vi "CvrtGrp2GXML.vi"(8 "error in (no error)":errorcluster, 11 "ChanGroups in":refnum<class "ChanGrp.lvclass">[](array[class])) -> (0 "error out":errorcluster, 1 "GXML Chans Oout":string[](array[string]), 3 "ChanGroups out":T1)   [LabVIEW 2018, in "Configuration Grandmaster.lvlib" / "ChanGrp.lvclass"]
uses:
  ChanGrp.lvclass
  Custom Ctrls/Master CfgXML/ge_XMLHdr_ChanGroups.ctl
  Custom Ctrls/Master Cfg/ge_GrpHdr.ctl
  Custom Ctrls/ge_MeasType.ctl
  ChanGrp.lvclass/ChanGrp.ctl
  Measurement Type Defs/VoltGroup.ctl
  Measurement Type Defs/VoltChan.ctl
  Measurements/Class Channel/ChanProps_TD.ctl
  Measurements/Class Voltage/VoltProps_TD.ctl
  Measurements/Class Voltage/Voltage.lvclass
  Measurement Type Defs/FreqGroup.ctl
  Measurement Type Defs/FreqChan.ctl
  Measurements/Class Frequency/FreqProps_TD.ctl
  Measurements/Class Frequency/Frequency.lvclass
  Measurement Type Defs/TachGroup.ctl
  Measurement Type Defs/TachChan.ctl
  Measurements/Class Tachometer/TachProps_TD.ctl
  Measurements/Class Tachometer/Tachometer.lvclass
  Measurement Type Defs/DynGroup.ctl
  Measurement Type Defs/DyanChan.ctl
  Measurements/Class Dynamic/DynamicProps_TD.ctl
  Measurements/Class Dynamic/Dynamic.lvclass
  Measurement Type Defs/StrainGroup.ctl
  Measurement Type Defs/StrainChan.ctl
  Measurements/Class Strain/StrainProps_TD.ctl
  Measurements/Class Strain/Strain.lvclass
  Measurement Type Defs/ThrmcplGroup.ctl
  Measurement Type Defs/ThrmcplChan.ctl
  Measurements/Class Thermocouple/ThrmcplProps_TD.ctl
  Measurements/Class Thermocouple/Thermocouple.lvclass
  Measurement Type Defs/RTDGroup.ctl
  Measurement Type Defs/RTDChan.ctl
  Measurements/Class RTD/RTDProps_TD.ctl
  Measurements/Class RTD/RTD.lvclass
  Measurement Type Defs/CurrentGroup.ctl
  Measurement Type Defs/CurrentChan.ctl
  Measurements/Class Current/CurrentProps_TD.ctl
  Measurements/Class Current/Current.lvclass
  Measurement Type Defs/ResGroup.ctl
  Measurement Type Defs/ResChan.ctl
  Measurements/Class Ressistance/ResProps_TD.ctl
  Measurements/Class Ressistance/Resistance.lvclass
  Measurements/Class Channel/Channel.lvclass
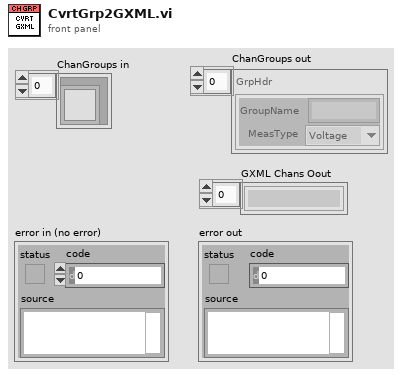
[diagram p1: front panel]
types:
  T1 = typedef "ge_XMLHdr_ChanGroups.ctl" = T2[]
  T2 = typedef "ge_GrpHdr.ctl" = cluster{"GroupName":string, "MeasType":T3}
  T3 = typedef "ge_MeasType.ctl" = enum16{"Voltage", "Frequency", "Tachometer", "Dynamic", "Thermocouple", "RTD", "Strain", "Current", "Resistance"}
  T4 = typedef "Configuration Grandmaster.lvlib/ChanGrp.lvclass/VoltGroup.ctl" = cluster{"GroupName":string, "MeasType":T3, "GroupMems":T5[]}
  T5 = typedef "Configuration Grandmaster.lvlib/ChanGrp.lvclass/VoltChan.ctl" = cluster{"ChanHdr":T6, "VoltChanCfg":T7}
  T6 = typedef "Measurement Channels.lvlib/Channel.lvclass/ChanProps_TD.ctl" = cluster{"ChanName":string, "ModbusAddr":string, "ToModBus":bool, "Alias":string, "Device":string, "Unit_EU":string, "Scale":dbl, "Offset":dbl}
  T7 = typedef "Measurement Channels.lvlib/Voltage.lvclass/VoltProps_TD.ctl" = cluster{"VRange":dbl, "Term Cfg":u16, "Coupling":u16}
  T8 = typedef "Configuration Grandmaster.lvlib/ChanGrp.lvclass/FreqGroup.ctl" = cluster{"GroupName":string, "MeasType":T3, "GroupMems":T9[]}
  T9 = typedef "Configuration Grandmaster.lvlib/ChanGrp.lvclass/FreqChan.ctl" = cluster{"ChanHdr":T6, "VoltChanCfg":T7, "FreqChanCfg":T10}
  T10 = typedef "Measurement Channels.lvlib/Frequency.lvclass/FreqProps_TD.ctl" = cluster{"Thresh":dbl, "Slope":u16, "Min EU":dbl}
  T11 = typedef "Configuration Grandmaster.lvlib/ChanGrp.lvclass/TachGroup.ctl" = cluster{"GroupName":string, "MeasType":T3, "GroupMems":T12[]}
  T12 = typedef "Configuration Grandmaster.lvlib/ChanGrp.lvclass/TachChan.ctl" = cluster{"ChanHdr":T6, "VoltChanCfg":T7, "FreqChanCfg":T10, "TachChanCfg":T13}
  T13 = typedef "Measurement Channels.lvlib/Tachometer.lvclass/TachProps_TD.ctl" = cluster{"PPR":dbl}
  T14 = typedef "Configuration Grandmaster.lvlib/ChanGrp.lvclass/DynGroup.ctl" = cluster{"GroupName":string, "MeasType":T3, "GroupMems":T15[]}
  T15 = typedef "Configuration Grandmaster.lvlib/ChanGrp.lvclass/DyanChan.ctl" = cluster{"ChanHdr":T6, "VoltChanCfg":T7, "DynChanCfg":T16}
  T16 = typedef "Measurement Channels.lvlib/Dynamic.lvclass/DynamicProps_TD.ctl" = cluster{"Sensitivity":dbl, "Iex":dbl, "dB":bool, "dB Ref":dbl, "Cal Mag":dbl, "Cal Units":u16}
  T17 = typedef "Configuration Grandmaster.lvlib/ChanGrp.lvclass/StrainGroup.ctl" = cluster{"GroupName":string, "MeasType":T3, "GroupMems":T18[]}
  T18 = typedef "Configuration Grandmaster.lvlib/ChanGrp.lvclass/StrainChan.ctl" = cluster{"ChanHdr":T6, "StrainChanCfg":T19}
  T19 = typedef "Measurement Channels.lvlib/Strain.lvclass/StrainProps_TD.ctl" = cluster{"Strain Mode":u16, "Vex":dbl, "Bridge Type":u16, "GF":dbl, "Gauge Res":i32, "Poisson":dbl, "Lead Res":dbl, "Init uStrain":dbl, "GAF":dbl, "Approx Max":dbl, "Approx Min":dbl}
  T20 = typedef "Configuration Grandmaster.lvlib/ChanGrp.lvclass/ThrmcplGroup.ctl" = cluster{"GroupName":string, "MeasType":T3, "GroupMems":T21[]}
  T21 = typedef "Configuration Grandmaster.lvlib/ChanGrp.lvclass/ThrmcplChan.ctl" = cluster{"ChanHdr":T6, "ThrmcplChanCfg":T22}
  T22 = typedef "Measurement Channels.lvlib/Thermocouple.lvclass/ThrmcplProps_TD.ctl" = cluster{"Units":u16, "Type":u16, "cjc source":u16, "cjc val":dbl, "Approx Max":dbl, "Approx Min":dbl}
  T23 = typedef "Configuration Grandmaster.lvlib/ChanGrp.lvclass/RTDGroup.ctl" = cluster{"GroupName":string, "MeasType":T3, "GroupMems":T24[]}
  T24 = typedef "Configuration Grandmaster.lvlib/ChanGrp.lvclass/RTDChan.ctl" = cluster{"ChanHdr":T6, "RTDChanCfg":T25}
  T25 = typedef "Measurement Channels.lvlib/RTD.lvclass/RTDProps_TD.ctl" = cluster{"Ro":u16, "Units":u16, "Type":u16, "WireCfg":u16, "Approx Max":dbl, "Approx Min":dbl}
  T26 = typedef "Configuration Grandmaster.lvlib/ChanGrp.lvclass/CurrentGroup.ctl" = cluster{"GroupName":string, "MeasType":T3, "GroupMems":T27[]}
  T27 = typedef "Configuration Grandmaster.lvlib/ChanGrp.lvclass/CurrentChan.ctl" = cluster{"ChanHdr":T6, "CurrentChanCfg":T28}
  T28 = typedef "CurrentProps_TD.ctl" = cluster{"IRange":dbl}
  T29 = typedef "Configuration Grandmaster.lvlib/ChanGrp.lvclass/ResGroup.ctl" = cluster{"GroupName":string, "MeasType":T3, "GroupMems":T30[]}
  T30 = typedef "Configuration Grandmaster.lvlib/ChanGrp.lvclass/ResChan.ctl" = cluster{"ChanHdr":T6, "ResChanCfg":T31}
  T31 = typedef "Measurement Channels.lvlib/Resistance.lvclass/ResProps_TD.ctl" = cluster{"ORange":u16, "WireCfg":u16}
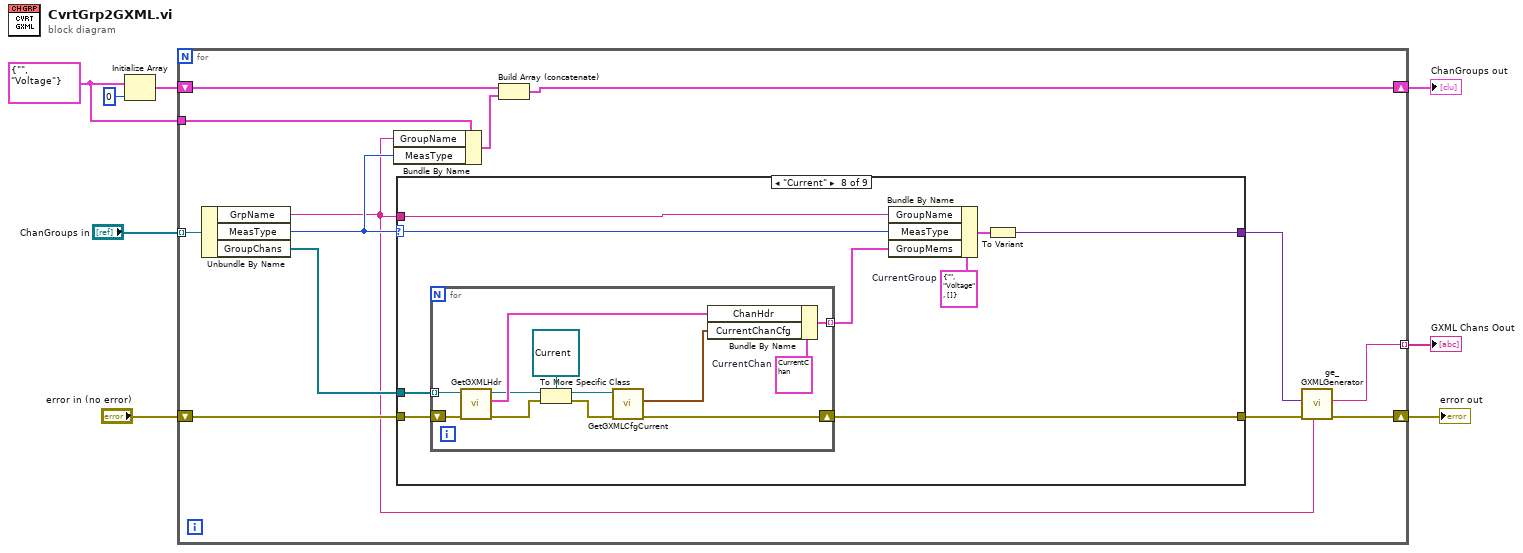
[diagram p0: block diagram]
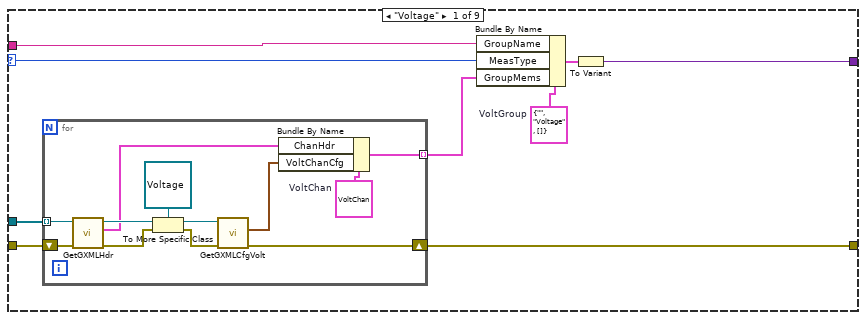
[diagram p2: hidden frame]
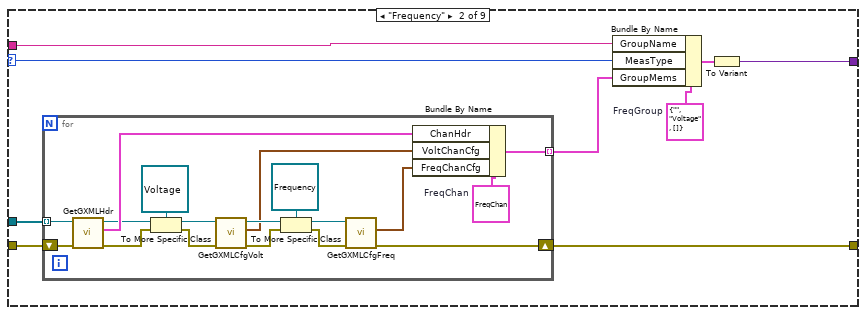
[diagram p3: hidden frame]
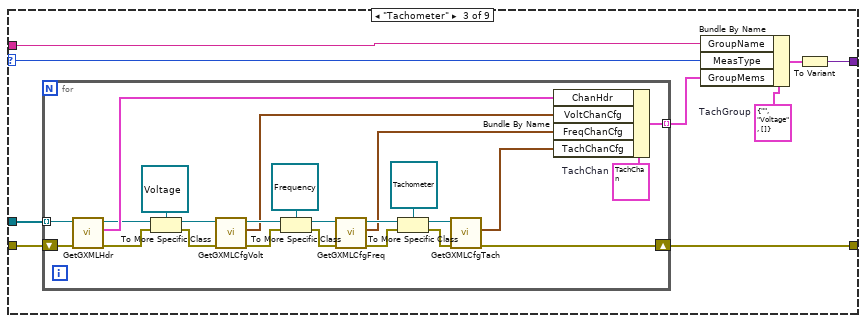
[diagram p4: hidden frame]
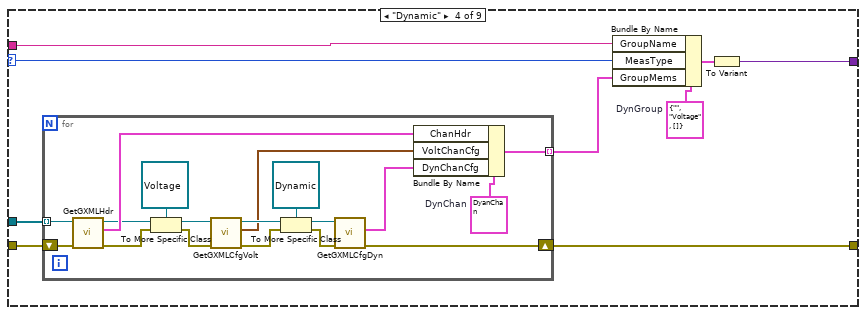
[diagram p5: hidden frame]
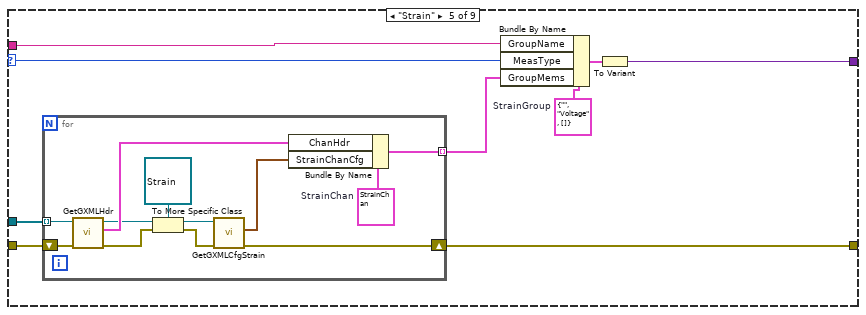
[diagram p6: hidden frame]
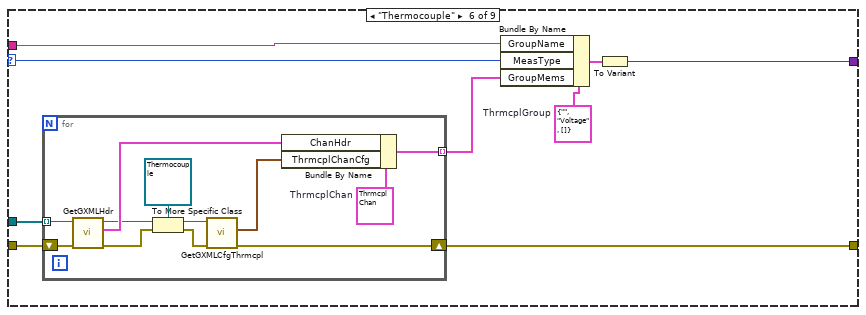
[diagram p7: hidden frame]
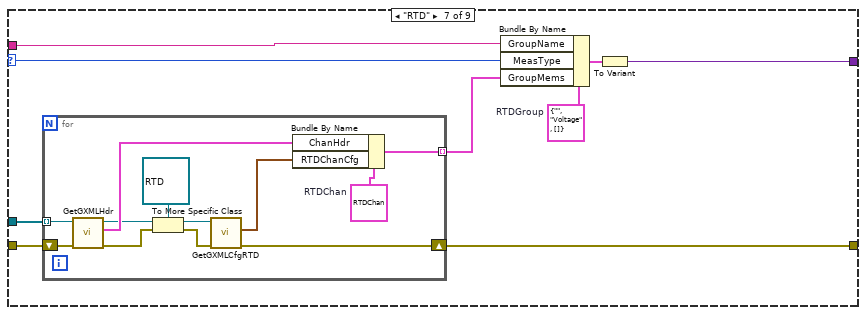
[diagram p8: hidden frame]
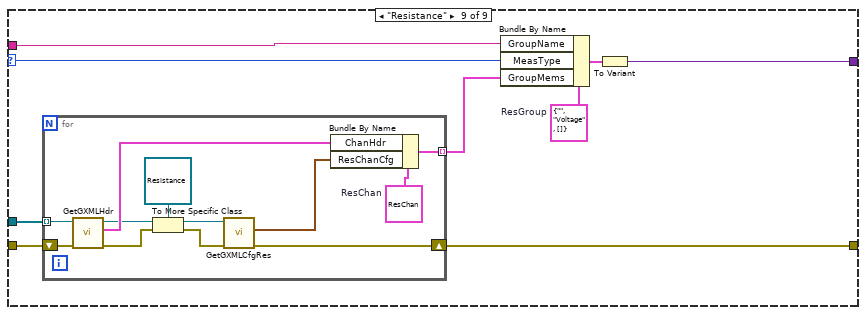
[diagram p9: hidden frame]
diagram:
  w1 = T2 {"GroupName"="", "MeasType"=enum."Voltage"} ("GrpHdr")
  n1 = Initialize Array(w1, 0 ("dimension size")) -> (w3:T2[])
  n2 = for {
    tunnel: "ChanGroups in" -> [w15] mode=indexing
    shift-right: [w21] -> w4
    shift-left: w3 -> [w17]
    shift-right: [w19] -> w7
    shift-left: "error in (no error)" -> [w14]
    tunnel: [w16] -> w8 mode=indexing
    tunnel: w1 -> [w10]
    n3 = Unbundle By Name(w15) -> ("GrpName"=w11:string, "MeasType"=w13:T3, "GroupChans"=w12:refnum<class "Channel.lvclass">[])
    n4 = Bundle By Name(cluster=w10, "GroupName"=w11, "MeasType"=w13) -> (w9:T2)
    n5 = case shown="\"Current\"" w13 {
      selector: w13 -> [w22 w44 w71 w104 w131 w152 w173 w194 w215]
      tunnel: w14 -> [w30 w51 w78 w111 w138 w159 w180 w201 w222]
      tunnel: w11 -> [w27 w49 w76 w109 w136 w157 w178 w199 w220]
      tunnel: [w25 w47 w74 w107 w134 w155 w176 w197 w218] -> w20
      tunnel: [w24 w46 w73 w106 w133 w154 w175 w196 w217] -> w18
      tunnel: w12 -> [w23 w45 w72 w105 w132 w153 w174 w195 w216]
      frame "Voltage" {
        w28 = T4 {"GroupName"="", "MeasType"=enum."Voltage", "GroupMems"=[]}  # VoltGroup
        n6 = for {
          tunnel: w23 -> [w42] mode=indexing
          tunnel: [w35] -> w26 mode=indexing
          shift-right: [w31] -> w25
          shift-left: w30 -> [w41]
          w36 = T5 {"ChanHdr"={"ChanName"="", "ModbusAddr"="", "ToModBus"=FALSE, "Alias"="", "Device"="", "Unit_EU"="", "Scale"=0.0, "Offset"=0.0}, "VoltChanCfg"={"VRange"=0.0, "Term Cfg"=0, "Coupling"=0}}  # VoltChan
          n7 = call "GetGXMLHdr.vi"("error in (no error)"=w41, "Channel in"=w42) -> ("error out"=w40:errorcluster, "ChanHdr"=w38:T6, "Channel out"=w39:refnum<class "Channel.lvclass">)  [unwired: 7 in]
          n8 = To More Specific Class(target class=refnum<class "Voltage.lvclass"> refnum ("Voltage.lvclass"), reference=w39, error in=w40) -> (specific class reference=w34:refnum<class "Voltage.lvclass">, error out=w33:errorcluster)
          n9 = call "GetGXMLCfgVolt.vi"("error in (no error)"=w33, "Voltage in"=w34) -> ("error out"=w31:errorcluster, "Voltage Cfg"=w32:T7)  [unwired: 7 in, 1 out]
          n10 = Bundle By Name(cluster=w36, "ChanHdr"=w38, "VoltChanCfg"=w32) -> (w35:T5)
        }
        n11 = Bundle By Name(cluster=w28, "GroupName"=w27, "MeasType"=w22, "GroupMems"=w26) -> (w29:T4)
        n12 = To Variant(anything=w29) -> (Variant=w24:variant)
      }
      frame "Frequency" {
        w43 = T8 {"GroupName"="", "MeasType"=enum."Voltage", "GroupMems"=[]}  # FreqGroup
        n13 = for {
          tunnel: w45 -> [w69] mode=indexing
          tunnel: [w66] -> w48 mode=indexing
          shift-right: [w63] -> w47
          shift-left: w51 -> [w68]
          w60 = T9 {"ChanHdr"={"ChanName"="", "ModbusAddr"="", "ToModBus"=FALSE, "Alias"="", "Device"="", "Unit_EU"="", "Scale"=0.0, "Offset"=0.0}, "VoltChanCfg"={"VRange"=0.0, "Term Cfg"=0, "Coupling"=0}, "FreqChanCfg"={"Thresh"=0.0, "Slope"=0, "Min EU"=0.0}}  # FreqChan
          n14 = call "GetGXMLHdr.vi"("error in (no error)"=w68, "Channel in"=w69) -> ("error out"=w55:errorcluster, "ChanHdr"=w67:T6, "Channel out"=w56:refnum<class "Channel.lvclass">)  [unwired: 7 in]
          n15 = To More Specific Class(target class=refnum<class "Voltage.lvclass"> refnum ("Voltage.lvclass"), reference=w56, error in=w55) -> (specific class reference=w58:refnum<class "Voltage.lvclass">, error out=w57:errorcluster)
          n16 = call "GetGXMLCfgVolt.vi"("error in (no error)"=w57, "Voltage in"=w58) -> ("error out"=w53:errorcluster, "Voltage Cfg"=w52:T7, "Voltage out"=w54:refnum<class "Voltage.lvclass">)  [unwired: 7 in]
          n17 = To More Specific Class(target class=refnum<class "Frequency.lvclass"> refnum ("Frequency.lvclass"), reference=w54, error in=w53) -> (specific class reference=w65:refnum<class "Frequency.lvclass">, error out=w64:errorcluster)
          n18 = call "GetGXMLCfgFreq.vi"("error in (no error)"=w64, "Freq in"=w65) -> ("error out"=w63:errorcluster, "FreqChanCfg"=w61:T10)  [unwired: 7 in, 1 out]
          n19 = Bundle By Name(cluster=w60, "ChanHdr"=w67, "VoltChanCfg"=w52, "FreqChanCfg"=w61) -> (w66:T9)
        }
        n20 = Bundle By Name(cluster=w43, "GroupName"=w49, "MeasType"=w44, "GroupMems"=w48) -> (w50:T8)
        n21 = To Variant(anything=w50) -> (Variant=w46:variant)
      }
      frame "Tachometer" {
        w70 = T11 {"GroupName"="", "MeasType"=enum."Voltage", "GroupMems"=[]}  # TachGroup
        n22 = for {
          tunnel: w72 -> [w102] mode=indexing
          tunnel: [w99] -> w75 mode=indexing
          shift-right: [w80] -> w74
          shift-left: w78 -> [w101]
          w87 = T12 {"ChanHdr"={"ChanName"="", "ModbusAddr"="", "ToModBus"=FALSE, "Alias"="", "Device"="", "Unit_EU"="", "Scale"=0.0, "Offset"=0.0}, "VoltChanCfg"={"VRange"=0.0, "Term Cfg"=0, "Coupling"=0}, "FreqChanCfg"={"Thresh"=0.0, "Slope"=0, "Min EU"=0.0}, "TachChanCfg"={"PPR"=0.0}}  # TachChan
          n23 = call "GetGXMLHdr.vi"("error in (no error)"=w101, "Channel in"=w102) -> ("error out"=w91:errorcluster, "ChanHdr"=w100:T6, "Channel out"=w92:refnum<class "Channel.lvclass">)  [unwired: 7 in]
          n24 = To More Specific Class(target class=refnum<class "Voltage.lvclass"> refnum ("Voltage.lvclass"), reference=w92, error in=w91) -> (specific class reference=w94:refnum<class "Voltage.lvclass">, error out=w93:errorcluster)
          n25 = call "GetGXMLCfgVolt.vi"("error in (no error)"=w93, "Voltage in"=w94) -> ("error out"=w89:errorcluster, "Voltage Cfg"=w88:T7, "Voltage out"=w90:refnum<class "Voltage.lvclass">)  [unwired: 7 in]
          n26 = To More Specific Class(target class=refnum<class "Frequency.lvclass"> refnum ("Frequency.lvclass"), reference=w90, error in=w89) -> (specific class reference=w98:refnum<class "Frequency.lvclass">, error out=w97:errorcluster)
          n27 = call "GetGXMLCfgFreq.vi"("error in (no error)"=w97, "Freq in"=w98) -> ("error out"=w85:errorcluster, "FreqChanCfg"=w83:T10, "Freq out"=w86:refnum<class "Frequency.lvclass">)  [unwired: 7 in]
          n28 = To More Specific Class(target class=refnum<class "Tachometer.lvclass"> refnum ("Tachometer.lvclass"), reference=w86, error in=w85) -> (specific class reference=w82:refnum<class "Tachometer.lvclass">, error out=w81:errorcluster)
          n29 = call "GetGXMLCfgTach.vi"("error in (no error)"=w81, "Tachometer in"=w82) -> ("error out"=w80:errorcluster, "TachChanCfg"=w79:T13)  [unwired: 7 in, 1 out]
          n30 = Bundle By Name(cluster=w87, "ChanHdr"=w100, "VoltChanCfg"=w88, "FreqChanCfg"=w83, "TachChanCfg"=w79) -> (w99:T12)
        }
        n31 = Bundle By Name(cluster=w70, "GroupName"=w76, "MeasType"=w71, "GroupMems"=w75) -> (w77:T11)
        n32 = To Variant(anything=w77) -> (Variant=w73:variant)
      }
      frame "Dynamic" {
        w103 = T14 {"GroupName"="", "MeasType"=enum."Voltage", "GroupMems"=[]}  # DynGroup
        n33 = for {
          tunnel: w105 -> [w129] mode=indexing
          tunnel: [w126] -> w108 mode=indexing
          shift-right: [w113] -> w107
          shift-left: w111 -> [w128]
          w118 = T15 {"ChanHdr"={"ChanName"="", "ModbusAddr"="", "ToModBus"=FALSE, "Alias"="", "Device"="", "Unit_EU"="", "Scale"=0.0, "Offset"=0.0}, "VoltChanCfg"={"VRange"=0.0, "Term Cfg"=0, "Coupling"=0}, "DynChanCfg"={"Sensitivity"=0.0, "Iex"=0.0, "dB"=FALSE, "dB Ref"=0.0, "Cal Mag"=0.0, "Cal Units"=0}}  # DynChan
          n34 = call "GetGXMLHdr.vi"("error in (no error)"=w128, "Channel in"=w129) -> ("error out"=w121:errorcluster, "ChanHdr"=w127:T6, "Channel out"=w122:refnum<class "Channel.lvclass">)  [unwired: 7 in]
          n35 = To More Specific Class(target class=refnum<class "Voltage.lvclass"> refnum ("Voltage.lvclass"), reference=w122, error in=w121) -> (specific class reference=w124:refnum<class "Voltage.lvclass">, error out=w123:errorcluster)
          n36 = call "GetGXMLCfgVolt.vi"("error in (no error)"=w123, "Voltage in"=w124) -> ("error out"=w119:errorcluster, "Voltage Cfg"=w117:T7, "Voltage out"=w120:refnum<class "Voltage.lvclass">)  [unwired: 7 in]
          n37 = To More Specific Class(target class=refnum<class "Dynamic.lvclass"> refnum ("Dynamic.lvclass"), reference=w120, error in=w119) -> (specific class reference=w115:refnum<class "Dynamic.lvclass">, error out=w114:errorcluster)
          n38 = call "GetGXMLCfgDyn.vi"("error in (no error)"=w114, "Dynamic in"=w115) -> ("error out"=w113:errorcluster, "DynChanCfg"=w112:T16)  [unwired: 7 in, 1 out]
          n39 = Bundle By Name(cluster=w118, "ChanHdr"=w127, "VoltChanCfg"=w117, "DynChanCfg"=w112) -> (w126:T15)
        }
        n40 = Bundle By Name(cluster=w103, "GroupName"=w109, "MeasType"=w104, "GroupMems"=w108) -> (w110:T14)
        n41 = To Variant(anything=w110) -> (Variant=w106:variant)
      }
      frame "Strain" {
        w130 = T17 {"GroupName"="", "MeasType"=enum."Voltage", "GroupMems"=[]}  # StrainGroup
        n42 = for {
          tunnel: w132 -> [w150] mode=indexing
          tunnel: [w147] -> w135 mode=indexing
          shift-right: [w140] -> w134
          shift-left: w138 -> [w149]
          w146 = T18 {"ChanHdr"={"ChanName"="", "ModbusAddr"="", "ToModBus"=FALSE, "Alias"="", "Device"="", "Unit_EU"="", "Scale"=0.0, "Offset"=0.0}, "StrainChanCfg"={"Strain Mode"=0, "Vex"=0.0, "Bridge Type"=0, "GF"=0.0, "Gauge Res"=0, "Poisson"=0.0, "Lead Res"=0.0, "Init uStrain"=0.0, "GAF"=0.0, "Approx Max"=0.0, "Approx Min"=0.0}}  # StrainChan
          n43 = call "GetGXMLHdr.vi"("error in (no error)"=w149, "Channel in"=w150) -> ("error out"=w145:errorcluster, "ChanHdr"=w148:T6, "Channel out"=w144:refnum<class "Channel.lvclass">)  [unwired: 7 in]
          n44 = To More Specific Class(target class=refnum<class "Strain.lvclass"> refnum ("Strain.lvclass"), reference=w144, error in=w145) -> (specific class reference=w141:refnum<class "Strain.lvclass">, error out=w142:errorcluster)
          n45 = call "GetGXMLCfgStrain.vi"("error in (no error)"=w142, "Strain in"=w141) -> ("error out"=w140:errorcluster, "StrainChanCfg"=w139:T19)  [unwired: 7 in, 1 out]
          n46 = Bundle By Name(cluster=w146, "ChanHdr"=w148, "StrainChanCfg"=w139) -> (w147:T18)
        }
        n47 = Bundle By Name(cluster=w130, "GroupName"=w136, "MeasType"=w131, "GroupMems"=w135) -> (w137:T17)
        n48 = To Variant(anything=w137) -> (Variant=w133:variant)
      }
      frame "Thermocouple" {
        w151 = T20 {"GroupName"="", "MeasType"=enum."Voltage", "GroupMems"=[]}  # ThrmcplGroup
        n49 = for {
          tunnel: w153 -> [w171] mode=indexing
          tunnel: [w168] -> w156 mode=indexing
          shift-right: [w161] -> w155
          shift-left: w159 -> [w170]
          w165 = T21 {"ChanHdr"={"ChanName"="", "ModbusAddr"="", "ToModBus"=FALSE, "Alias"="", "Device"="", "Unit_EU"="", "Scale"=0.0, "Offset"=0.0}, "ThrmcplChanCfg"={"Units"=0, "Type"=0, "cjc source"=0, "cjc val"=0.0, "Approx Max"=0.0, "Approx Min"=0.0}}  # ThrmcplChan
          n50 = call "GetGXMLHdr.vi"("error in (no error)"=w170, "Channel in"=w171) -> ("error out"=w167:errorcluster, "ChanHdr"=w169:T6, "Channel out"=w166:refnum<class "Channel.lvclass">)  [unwired: 7 in]
          n51 = To More Specific Class(target class=refnum<class "Thermocouple.lvclass"> refnum ("Thermocouple.lvclass"), reference=w166, error in=w167) -> (specific class reference=w163:refnum<class "Thermocouple.lvclass">, error out=w162:errorcluster)
          n52 = call "GetGXMLCfgThrmcpl.vi"("error in (no error)"=w162, "Thermocouple in"=w163) -> ("error out"=w161:errorcluster, "ThrmcplChanCfg"=w160:T22)  [unwired: 7 in, 1 out]
          n53 = Bundle By Name(cluster=w165, "ChanHdr"=w169, "ThrmcplChanCfg"=w160) -> (w168:T21)
        }
        n54 = Bundle By Name(cluster=w151, "GroupName"=w157, "MeasType"=w152, "GroupMems"=w156) -> (w158:T20)
        n55 = To Variant(anything=w158) -> (Variant=w154:variant)
      }
      frame "RTD" {
        w172 = T23 {"GroupName"="", "MeasType"=enum."Voltage", "GroupMems"=[]}  # RTDGroup
        n56 = for {
          tunnel: w174 -> [w192] mode=indexing
          tunnel: [w189] -> w177 mode=indexing
          shift-right: [w181] -> w176
          shift-left: w180 -> [w191]
          w185 = T24 {"ChanHdr"={"ChanName"="", "ModbusAddr"="", "ToModBus"=FALSE, "Alias"="", "Device"="", "Unit_EU"="", "Scale"=0.0, "Offset"=0.0}, "RTDChanCfg"={"Ro"=0, "Units"=0, "Type"=0, "WireCfg"=0, "Approx Max"=0.0, "Approx Min"=0.0}}  # RTDChan
          n57 = call "GetGXMLHdr.vi"("error in (no error)"=w191, "Channel in"=w192) -> ("error out"=w188:errorcluster, "ChanHdr"=w190:T6, "Channel out"=w187:refnum<class "Channel.lvclass">)  [unwired: 7 in]
          n58 = To More Specific Class(target class=refnum<class "RTD.lvclass"> refnum ("RTD.lvclass"), reference=w187, error in=w188) -> (specific class reference=w184:refnum<class "RTD.lvclass">, error out=w182:errorcluster)
          n59 = call "GetGXMLCfgRTD.vi"("error in (no error)"=w182, "RTD in"=w184) -> ("error out"=w181:errorcluster, "RTDChanCfg"=w183:T25)  [unwired: 7 in, 1 out]
          n60 = Bundle By Name(cluster=w185, "ChanHdr"=w190, "RTDChanCfg"=w183) -> (w189:T24)
        }
        n61 = Bundle By Name(cluster=w172, "GroupName"=w178, "MeasType"=w173, "GroupMems"=w177) -> (w179:T23)
        n62 = To Variant(anything=w179) -> (Variant=w175:variant)
      }
      frame "Current" {
        w193 = T26 {"GroupName"="", "MeasType"=enum."Voltage", "GroupMems"=[]}  # CurrentGroup
        n63 = for {
          tunnel: w195 -> [w213] mode=indexing
          tunnel: [w210] -> w198 mode=indexing
          shift-right: [w202] -> w197
          shift-left: w201 -> [w212]
          w206 = T27 {"ChanHdr"={"ChanName"="", "ModbusAddr"="", "ToModBus"=FALSE, "Alias"="", "Device"="", "Unit_EU"="", "Scale"=0.0, "Offset"=0.0}, "CurrentChanCfg"={"IRange"=0.0}}  # CurrentChan
          n64 = call "GetGXMLHdr.vi"("error in (no error)"=w212, "Channel in"=w213) -> ("error out"=w209:errorcluster, "ChanHdr"=w211:T6, "Channel out"=w208:refnum<class "Channel.lvclass">)  [unwired: 7 in]
          n65 = To More Specific Class(target class=refnum<class "Current.lvclass"> refnum ("Current.lvclass"), reference=w208, error in=w209) -> (specific class reference=w205:refnum<class "Current.lvclass">, error out=w204:errorcluster)
          n66 = call "GetGXMLCfgCurrent.vi"("error in (no error)"=w204, "Current in"=w205) -> ("error out"=w202:errorcluster, "CurrentChanCfg"=w203:T28)  [unwired: 7 in, 1 out]
          n67 = Bundle By Name(cluster=w206, "ChanHdr"=w211, "CurrentChanCfg"=w203) -> (w210:T27)
        }
        n68 = Bundle By Name(cluster=w193, "GroupName"=w199, "MeasType"=w194, "GroupMems"=w198) -> (w200:T26)
        n69 = To Variant(anything=w200) -> (Variant=w196:variant)
      }
      frame "Resistance" {
        w214 = T29 {"GroupName"="", "MeasType"=enum."Voltage", "GroupMems"=[]}  # ResGroup
        n70 = for {
          tunnel: w216 -> [w234] mode=indexing
          tunnel: [w231] -> w219 mode=indexing
          shift-right: [w223] -> w218
          shift-left: w222 -> [w233]
          w227 = T30 {"ChanHdr"={"ChanName"="", "ModbusAddr"="", "ToModBus"=FALSE, "Alias"="", "Device"="", "Unit_EU"="", "Scale"=0.0, "Offset"=0.0}, "ResChanCfg"={"ORange"=0, "WireCfg"=0}}  # ResChan
          n71 = call "GetGXMLHdr.vi"("error in (no error)"=w233, "Channel in"=w234) -> ("error out"=w230:errorcluster, "ChanHdr"=w232:T6, "Channel out"=w229:refnum<class "Channel.lvclass">)  [unwired: 7 in]
          n72 = To More Specific Class(target class=refnum<class "Resistance.lvclass"> refnum ("Resistance.lvclass"), reference=w229, error in=w230) -> (specific class reference=w226:refnum<class "Resistance.lvclass">, error out=w225:errorcluster)
          n73 = call "GetGXMLCfgRes.vi"("error in (no error)"=w225, "Resistance in"=w226) -> ("error out"=w223:errorcluster, "ResChanCfg"=w224:T31)  [unwired: 7 in, 1 out]
          n74 = Bundle By Name(cluster=w227, "ChanHdr"=w232, "ResChanCfg"=w224) -> (w231:T30)
        }
        n75 = Bundle By Name(cluster=w214, "GroupName"=w220, "MeasType"=w215, "GroupMems"=w219) -> (w221:T29)
        n76 = To Variant(anything=w221) -> (Variant=w217:variant)
      }
    }
    n77 = Build Array (concatenate)(w17, w9) -> (w21:T2[])
    n78 = call "ge_GXMLGenerator.vi"("String ID"=w11, "error in"=w20, "Variant"=w18) -> ("error out"=w19:errorcluster, "XML String Out"=w16:string)  [unwired: 7 in]
  }
  "GXML Chans Oout" <- w8
  "error out" <- w7
  "ChanGroups out" <- w4
